vi "Subvi_VoltageRamping_Teleop.vi"(8 "error in (no error)":errorcluster, 10 "threshold":dbl=0.1 format="%#_13g", 11 "VoltageIn":dbl) -> (0 "error out":errorcluster, 3 "voltage out":dbl)   [LabVIEW 2017]
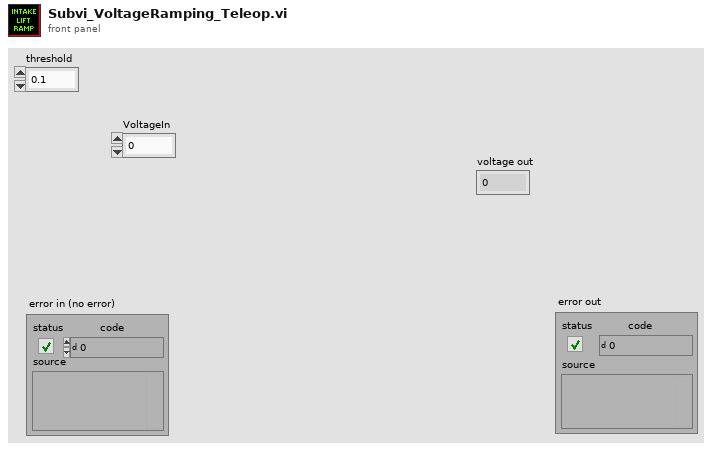
[diagram p1: front panel]
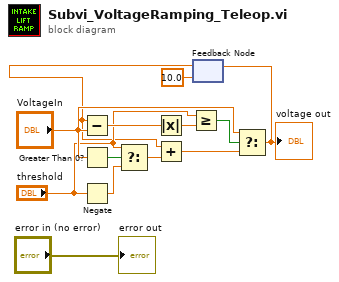
[diagram p0: block diagram]
diagram:
  n1 = Greater Than 0?(x="VoltageIn") -> (x > 0?=w8:bool)
  n2 = Negate(x="threshold") -> (-x=w6:dbl)
  n3 = Select(t="threshold", s=w8, f=w6) -> (s? t:f=w5:dbl)
  n4 = feedback #1(10.0 ("VoltageIn")) -> (w3:dbl)
  n5 = Subtract(x=w3, y="VoltageIn") -> (x-y=w12:dbl)
  n6 = Absolute Value(x=w12) -> (abs(x)=w11:dbl)
  n7 = Add(x=w3, y=w5) -> (x+y=w4:dbl)
  n8 = Greater Or Equal?(x="threshold", y=w11) -> (x >= y?=w10:bool)
  n9 = Select(t="VoltageIn", s=w10, f=w4) -> (s? t:f=w13:dbl)
  "voltage out" <- w13
  n10 = feedback-in #1(w13) -> ()
  "error out" <- "error in (no error)"
